vi "Generate Config Path.vi"(8 "error in":errorcluster, 11 "Philips UI in":refnum<class "Flex UI.lvclass">) -> (0 "error out":errorcluster, 2 "Config Path":path, 3 "Philips UI out":refnum<class "Flex UI.lvclass">)   [LabVIEW 2014, in "Flex UI.lvclass"]
uses:
  Flex UI.lvclass
  <vilib>/Utility/sysdir.llb/System Directory Type.ctl
  Flex UI.lvclass/Flex UI.ctl
  <userlib>/_OpenG.lib/file/file.llb/Build Path - Traditional__ogtk.vi
  <userlib>/_OpenG.lib/file/file.llb/Strip Path Extension - String__ogtk.vi
  <userlib>/_OpenG.lib/file/file.llb/Convert File Extension (String)__ogtk.vi
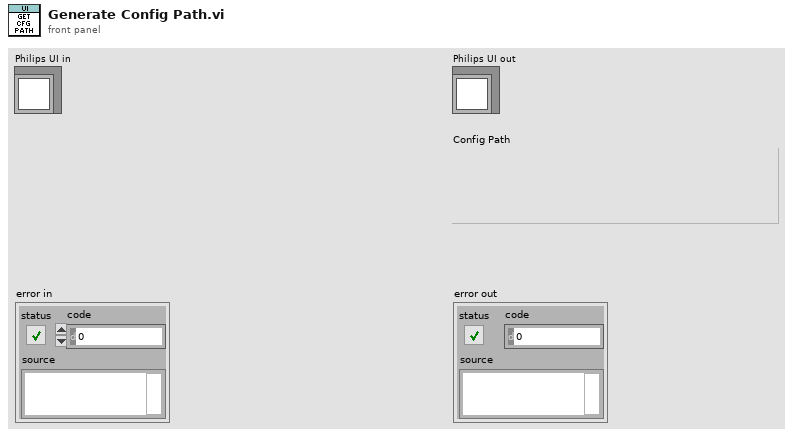
[diagram p1: front panel]
types:
  T1 = typedef "System Directory Type.ctl" = i32
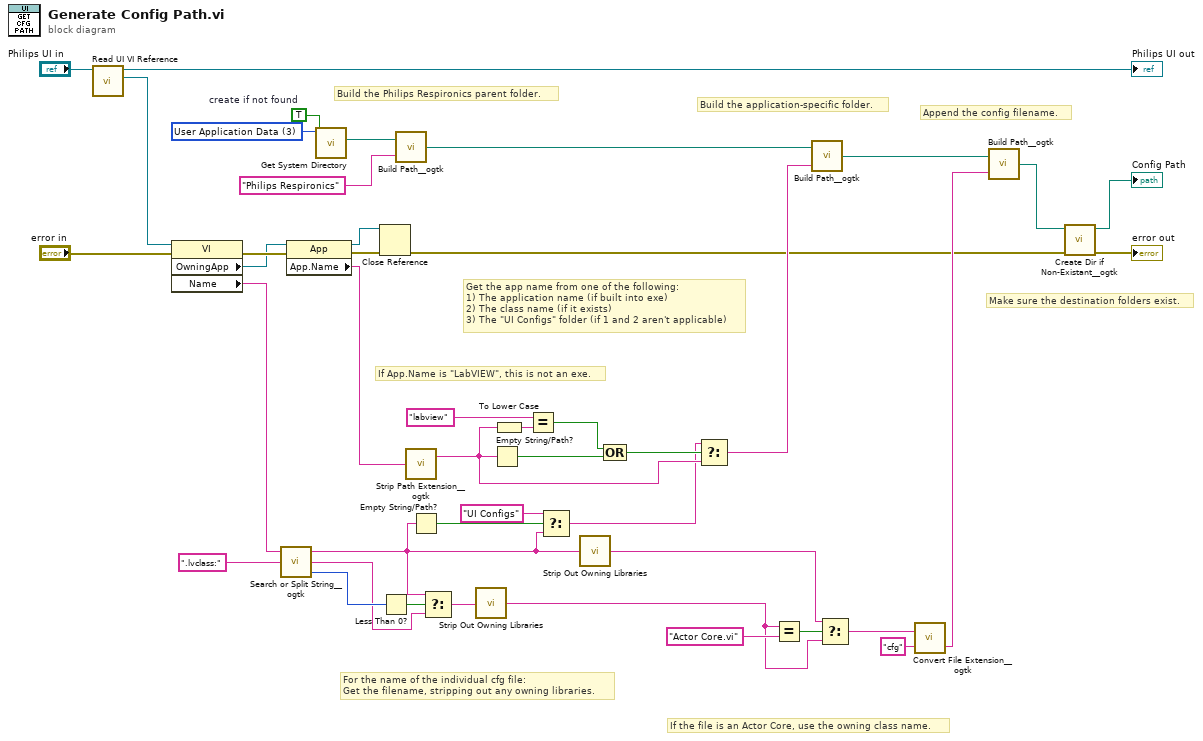
[diagram p0: block diagram]
diagram:
  w30 = TRUE  # create if not found
  w29 = T1 3 items=["User Home"=0, "User Desktop"=1, "User Documents"=2, "User Application Data"=3, "User Preferences"=4, "User Temporary"=5, "Public Documents"=6, "Public Application Data"=7, "Public Preferences"=8, "Public Cache"=13, "System Core Libraries"=9, "System Installed Libraries"=10, "Application Files"=11, "Boot Volume Root"=12] ("system directory type")
  # "If the file is an Actor Core, use the owning class name."
  # "If App.Name is \"LabVIEW\", this is not an exe."
  # "Make sure the destination folders exist."
  # "Append the config filename."
  # "For the name of the individual cfg file:\nGet the filename, stripping out any owning libraries."
  # "Get the app name from one of the following:\n1) The application name (if built into exe)\n2) The class name (if it exists)\n3) The \"UI Configs\" folder (if 1 and 2 aren't applicable)"
  # "Build the application-specific folder."
  # "Build the Philips Respironics parent folder."
  n1 = call "Read UI VI Reference.vi"("Philips UI in"="Philips UI in") -> ("UI VI Reference"=w11:refnum<vi>, "Philips UI out"=→"Philips UI out":refnum<class "Flex UI.lvclass">)  [unwired: 9 in]
  n2 = property class="VI"(reference=w11, error in="error in") -> (error out=w31:errorcluster, "OwningApp"=w25:refnum<vi>, "Name"=w2:string)  [unwired: 1 out]
  n3 = call <userlib>:"Search or Split String__ogtk.vi"("search string/char (-)"=".lvclass:", "string"=w2) -> ("offset after match"=w43:i32, "substring after match"=w34:string, "substring before match"=w6:string)  [unwired: 1 in]
  n4 = property class="App"(reference=w25, error in=w31) -> (reference out=w12:refnum<vi>, error out=w16:errorcluster, "App.Name"=w1:string)
  n5 = call <vilib>:"Get System Directory.vi"("create directory if not found? (F)"=w30, "system directory type"=w29) -> ("system directory"=w35:path)  [unwired: 9 in]
  n6 = Close Reference(reference=w12, error in (no error)=w16) -> (error out=w13:errorcluster)
  n7 = Less Than 0?(x=w43) -> (x < 0?=w33:bool)
  n8 = call-poly <userlib>:"Build Path__ogtk.vi"("name or relative path"="Philips Respironics", "base path"=w35) -> ("appended path"=w37:path)
  n9 = call-poly <userlib>:"Strip Path Extension__ogtk.vi"("path"=w1) -> ("root"=w18:string)  [unwired: 1 out]
  n10 = Empty String/Path?(string/path=w6) -> (empty?=w38:bool)
  n11 = Select(t=w6, s=w33, f=w34) -> (s? t:f=w8:string)
  n12 = call "Strip Out Owning Libraries.vi"("Original Name"=w8) -> ("Name w/o Libraries"=w5:string)
  n13 = Empty String/Path?(string/path=w18) -> (empty?=w20:bool)
  n14 = To Lower Case(string=w18) -> (all lower case string=w22:string)
  n15 = Equal?(x="labview", y=w22) -> (x = y?=w21:bool)
  n16 = Select(t="UI Configs", s=w38, f=w6) -> (s? t:f=w7:string)
  n17 = call "Strip Out Owning Libraries.vi"("Original Name"=w6) -> ("Name w/o Libraries"=w4:string)
  n18 = Compound Arithmetic op=OR(w21, w20) -> (w19:bool)
  n19 = Select(t=w7, s=w19, f=w18) -> (s? t:f=w24:string)
  n20 = Equal?(x=w5, y="Actor Core.vi") -> (x = y?=w9:bool)
  n21 = call-poly <userlib>:"Build Path__ogtk.vi"("name or relative path"=w24, "base path"=w37) -> ("appended path"=w40:path)
  n22 = Select(t=w4, s=w9, f=w5) -> (s? t:f=w3:string)
  n23 = call-poly <userlib>:"Convert File Extension__ogtk.vi"("new ending (none)"="cfg", "file name"=w3) -> ("prev ending"=w42:string)  [unwired: 1 out]
  n24 = call-poly <userlib>:"Build Path__ogtk.vi"("name or relative path"=w42, "base path"=w40) -> ("appended path"=w14:path)
  n25 = call <userlib>:"Create Dir if Non-Existant__ogtk.vi"("error in (no error)"=w13, "Directory Path"=w14) -> ("error out"=→"error out":errorcluster, "dup Directory Path"=→"Config Path":path)  [unwired: 7 in, 1 out]
